vi "String Delineator.vi"(6 "Ignore Empty Strings? (T)":bool=TRUE, 7 "Delineator \"&\"":string="&", 8 "error in (no error)":errorcluster, 9 "Array of Strings":string[](array[string]), 10 "Base String":string) -> (0 "error in (no error)":errorcluster, 2 "New String":string)   [LabVIEW 2012]
doc: "Takes a base string and appends each element of the string array separated by the delineator.\n\ni.e. \n\nBase URL = \"http://url.com/q=\"\nDelineator = \"&\"\nString Array = {\"one\",\"two\",\"three\"}\n\nbecomes\n\n\"http://url.com/q=one&two&three\"\n\nThis is useful for constructing compound URLs"
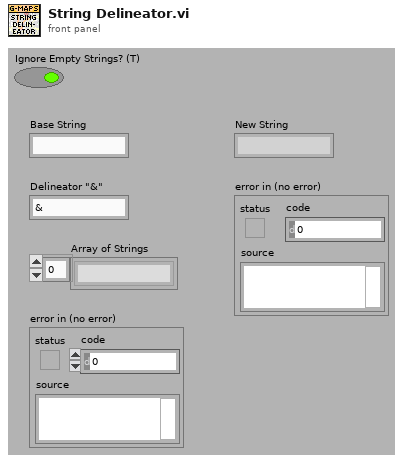
[diagram p1: front panel]
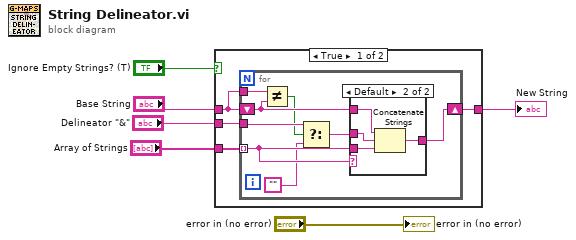
[diagram p0: block diagram]
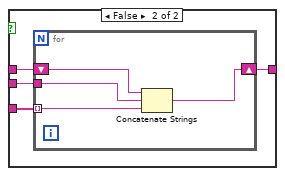
[diagram p3: hidden frame]
diagram:
  n1 = case shown="True" "Ignore Empty Strings? (T)" {
    tunnel: [w10 w27] -> w6
    tunnel: "Base String" -> [w7 w26]
    tunnel: "Delineator \"&\"" -> [w9 w25]
    tunnel: "Array of Strings" -> [w8 w24]
    frame True {
      n2 = for {
        tunnel: w8 -> [w17] mode=indexing
        shift-right: [w18] -> w10
        shift-left: w7 -> [w13]
        tunnel: w9 -> [w16]
        tunnel: w7 -> [w12]
        n3 = Not Equal?(x=w12, y=w13) -> (x != y?=w11:bool)
        n4 = Select(t=w16, s=w11, f="") -> (s? t:f=w15:string)
        n5 = case shown="Default" w17 {
          tunnel: w17 -> [_ w23]
          tunnel: [w19 w22] -> w18
          tunnel: w13 -> [w19 w21]
          tunnel: w15 -> [_ w20]
          frame "" {
          }
          frame Default {
            n6 = Concatenate Strings(w21, w20, w23) -> (w22:string)
          }
        }
      }
    }
    frame False {
      n7 = for {
        tunnel: w24 -> [w28] mode=indexing
        shift-right: [w31] -> w27
        shift-left: w26 -> [w30]
        tunnel: w25 -> [w29]
        n8 = Concatenate Strings(w30, w29, w28) -> (w31:string)
      }
    }
  }
  "New String" <- w6
  "error in (no error)" <- "error in (no error)"
